vi "ZK Create MB.vi"() -> ()   [LabVIEW 2016, in "质控单元V1.lvlib"]
uses:
  <vilib>/Plasmionique/MB Master/MB_Master_Serial/MB_Master_Serial.lvclass
  D:/Program Files (x86)/National Instruments/LabVIEW 2016/vi.lib/Plasmionique/MB Master/MB_Master/MB_Master.lvclass
  <vilib>/Plasmionique/MB Master/MB_Master_TCP/MB_Master_TCP.lvclass
  <vilib>/Plasmionique/MB Master/MB_Master/MB_Master.lvclass
panel:
  out "auto connected":bool=TRUE
  out "error out":errorcluster
  out "Connected":bool
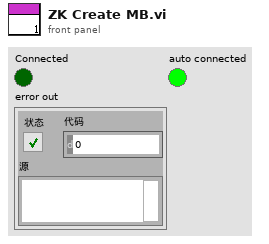
[diagram p1: front panel]
types:
  T1 = cluster{"baud rate (bps)":u32, "stop bits":u16, "parity":u16, "flow control":u16, "timeout":u32, "retries":i32}
  T2 = typedef "质控单元V1.lvlib/质控slave id.ctl" = enum16{"null", "氨氮", "总磷", "CODMn", "CODCr", "总氮"}
  T3 = cluster{"氨氮":bool, "总磷":bool, "总氮":bool, "CODMn":bool, "CODCr":bool, "氨氮总磷":bool, "总磷总氮":bool}
  T4 = typedef "质控单元V1.lvlib/质控仪器状态显示.ctl" = cluster{"运行模式":string, "运行状态":string, "液位状态":string, "告警状态":string, "加标体积":string}
  T5 = typedef "质控单元V1.lvlib/质控仪器状态.ctl" = cluster{"运行状态":T6, "加标体积":sgl, "NC":dbl, "液位状态":enum16{"无感应", "有感应"}, "告警状态":enum16{"无告警", "超时告警"}}
  T6 = typedef "质控单元V1.lvlib/质控运行状态.ctl" = enum16{"待机", "润洗", "进样", "加标", "排液", "搅拌", "超时告警"}
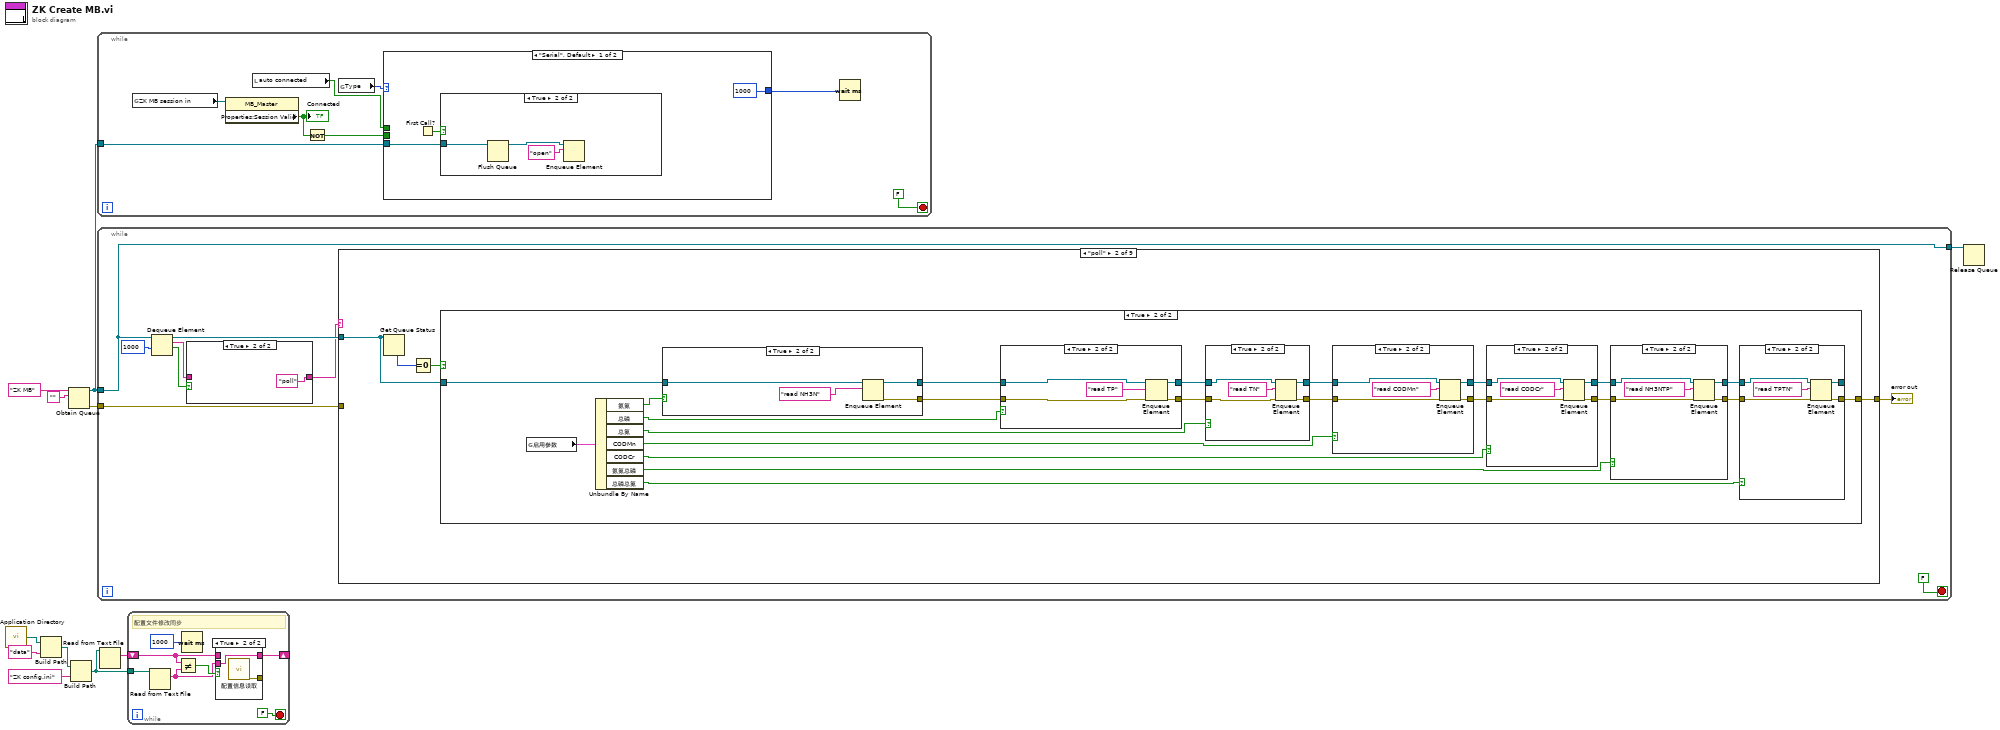
[diagram p0: block diagram]
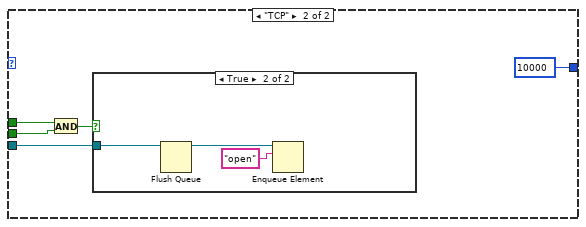
[diagram p4: hidden frame]
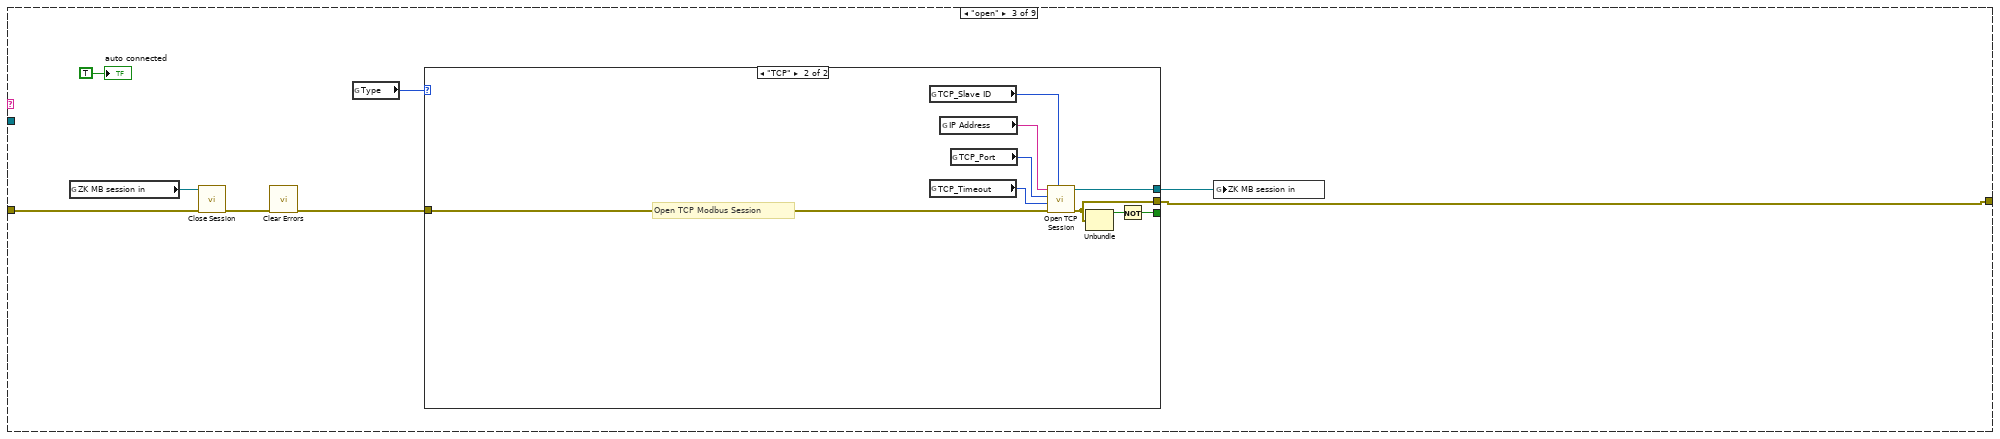
[diagram p16: hidden frame]
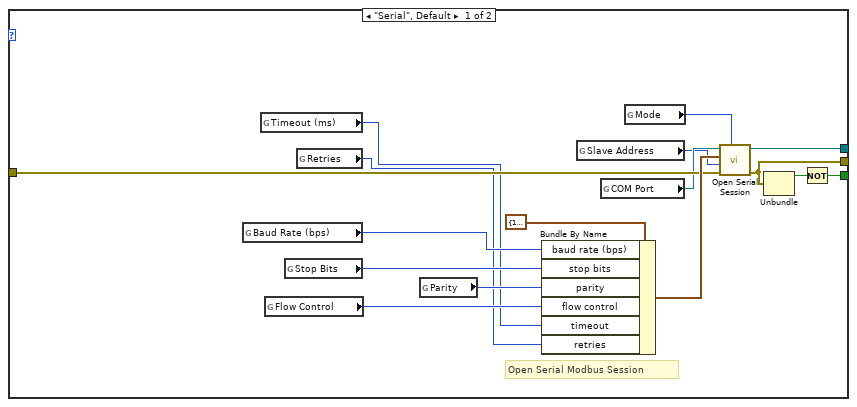
[diagram p17: hidden frame]
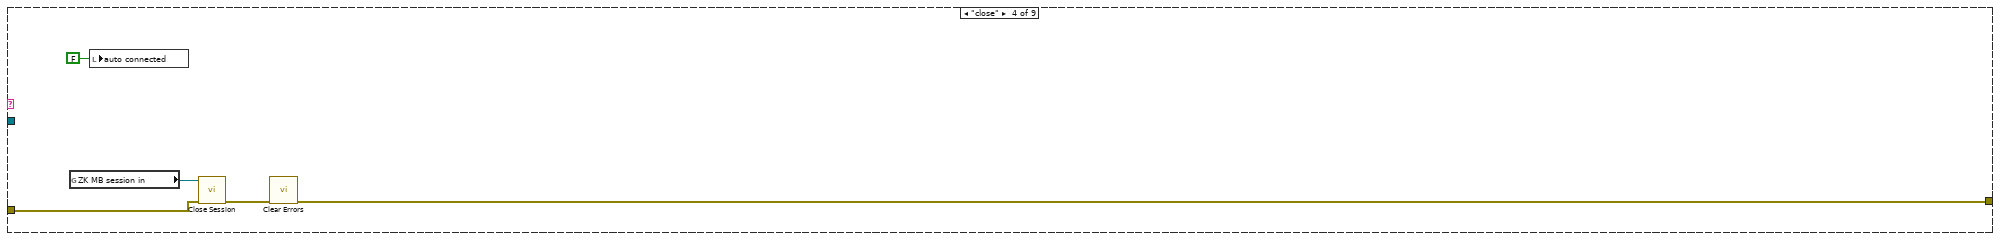
[diagram p18: hidden frame]
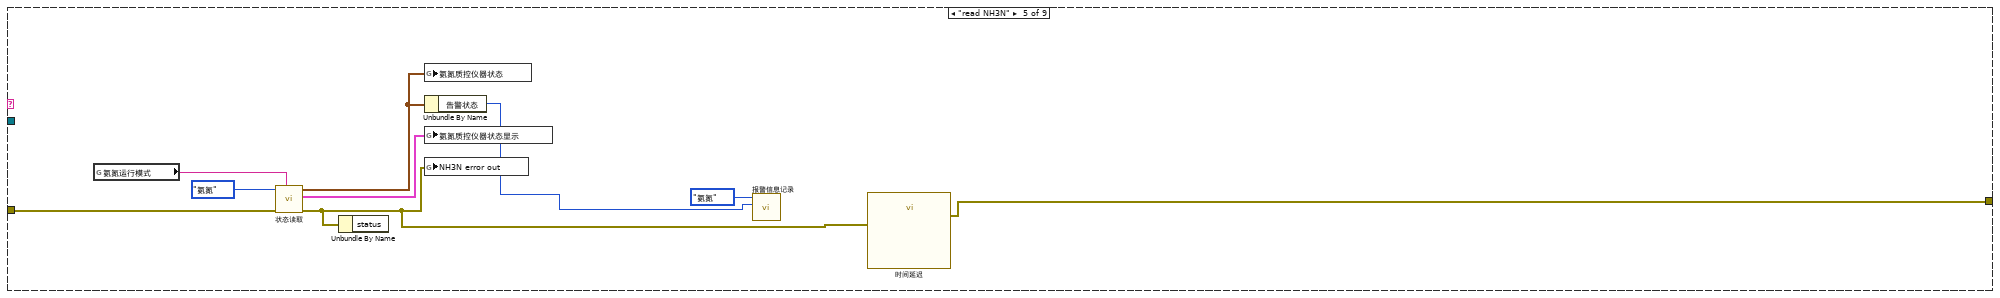
[diagram p19: hidden frame]
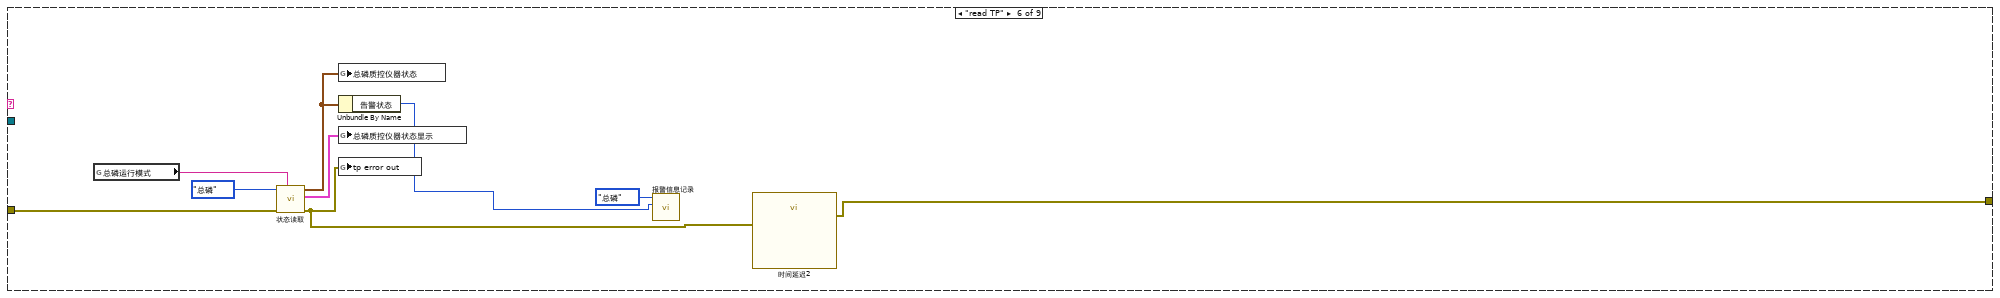
[diagram p20: hidden frame]
diagram:
  n1 = call <vilib>:"Application Directory.vi"() -> ("Application Directory"=w6:path)
  n2 = Build Path(base path=w6, name or relative path="data" ("名称或相对路径")) -> (appended path=w3:path)
  n3 = Obtain Queue(name (unnamed)="ZK MB" ("名称（未命名）"), element data type="") -> (queue out=w9:refnum<queue>, error out=w7:errorcluster)  [unwired: 3 in, 1 out]
  n4 = Build Path(base path=w3, name or relative path="ZK config.ini" ("名称或相对路径")) -> (appended path=w1:path)
  n5 = while {
    tunnel: w9 -> [w18]
    stop <- FALSE stop-if-true
    n6 = global read "ZK非断电保存全局变量.vi" "ZK MB session in"() -> (w15:refnum<class "MB_Master.lvclass">)
    n7 = property class="MB_Master"(reference=w15) -> ("Properties:Session Valid"=w14:bool)  [unwired: 1 in, 2 out]
    "Connected" <- w14
    n8 = local read "auto connected"() -> (w13:bool)
    n9 = Not(x=w14) -> (.not. x?=w12:bool)
    n10 = global read "ZK断电保存全局变量.vi" "Type"() -> (w19:enum16{"Serial", "TCP"})
    n11 = case shown="\"Serial\", Default" w19 {
      tunnel: w18 -> [w22 w30]
      tunnel: [u32 1000 ("等待时间（毫秒）") u32 10000 ("等待时间（毫秒）")] -> w16
      tunnel: w12 -> [_ w28]
      tunnel: w13 -> [_ w26]
      frame "Serial", Default {
        n12 = First Call?() -> (First Call?: T/F=w21:bool)
        n13 = case shown="True" w21 {
          tunnel: w22 -> [_ w25]
          frame False {
          }
          frame True {
            n14 = Flush Queue(queue=w25) -> (queue out=w23:refnum<queue>)  [unwired: 1 in, 2 out]
            n15 = Enqueue Element(queue=w23, element="open") -> ()  [unwired: 2 in, 3 out]
          }
        }
      }
      frame "TCP" {
        n16 = And(x=w26, y=w28) -> (x .and. y?=w27:bool)
        n17 = case shown="True" w27 {
          tunnel: w30 -> [_ w32]
          frame False {
          }
          frame True {
            n18 = Flush Queue(queue=w32) -> (queue out=w31:refnum<queue>)  [unwired: 1 in, 2 out]
            n19 = Enqueue Element(queue=w31, element="open") -> ()  [unwired: 2 in, 3 out]
          }
        }
      }
    }
    n20 = Wait (ms)(milliseconds to wait=w16) -> ()  [unwired: 1 out]
  }
  n21 = while {
    tunnel: w9 -> [w39]
    tunnel: [w39] -> w8
    tunnel: w7 -> [w34]
    stop <- FALSE stop-if-true
    n22 = Dequeue Element(queue=w39, timeout in ms (-1)=1000 ("超时毫秒(-1)")) -> (queue out=w40:refnum<queue>, element=w36:string, timed out?=w37:bool)  [unwired: 1 in, 1 out]
    n23 = case shown="True" w37 {
      tunnel: w36 -> [w43 _]
      tunnel: [w43 "poll"] -> w35
      frame False {
      }
      frame True {
      }
    }
    n24 = case shown="\"poll\"" w35 {
      tunnel: [w45 w49 w121 w154 w163 w173 w182 w190 w199] -> w41
      tunnel: w34 -> [w45 _ w120 w155 w165 w174 w183 w192 w201]
      tunnel: w40 -> [_ w48 _ _ _ _ _ _ _]
      frame Default {
      }
      frame "poll" {
        n25 = Get Queue Status(queue=w48) -> (# elements in queue=w47:i32)  [unwired: 2 in, 7 out]
        n26 = Equal To 0?(x=w47) -> (x = 0?=w46:bool)
        n27 = case shown="True" w46 {
          tunnel: [_ w55] -> w49
          tunnel: w48 -> [_ w50]
          frame False {
          }
          frame True {
            n28 = global read "ZK断电保存全局变量.vi" "启用参数"() -> (w63:T3)
            n29 = Unbundle By Name(w63) -> ("氨氮"=w62:bool, "总磷"=w61:bool, "总氮"=w60:bool, "CODMn"=w54:bool, "CODCr"=w53:bool, "氨氮总磷"=w52:bool, "总磷总氮"=w51:bool)
            n30 = case shown="True" w62 {
              tunnel: w50 -> [w114 w118]
              tunnel: [w114 w117] -> w71
              tunnel: [_ w116] -> w70
              frame False {
              }
              frame True {
                n31 = Enqueue Element(queue=w118, element="read NH3N") -> (queue out=w117:refnum<queue>, error out=w116:errorcluster)  [unwired: 2 in, 1 out]
              }
            }
            n32 = case shown="True" w61 {
              tunnel: w71 -> [w108 w113]
              tunnel: w70 -> [w107 w112]
              tunnel: [w108 w110] -> w69
              tunnel: [w107 w109] -> w66
              frame False {
              }
              frame True {
                n33 = Enqueue Element(queue=w113, element="read TP", error in (no error)=w112) -> (queue out=w110:refnum<queue>, error out=w109:errorcluster)  [unwired: 1 in, 1 out]
              }
            }
            n34 = case shown="True" w60 {
              tunnel: w69 -> [w101 w105]
              tunnel: [w101 w104] -> w59
              tunnel: w66 -> [w100 w103]
              tunnel: [w100 w102] -> w58
              frame False {
              }
              frame True {
                n35 = Enqueue Element(queue=w105, element="read TN", error in (no error)=w103) -> (queue out=w104:refnum<queue>, error out=w102:errorcluster)  [unwired: 1 in, 1 out]
              }
            }
            n36 = case shown="True" w54 {
              tunnel: w59 -> [w80 w84]
              tunnel: [w80 w83] -> w67
              tunnel: w58 -> [w79 w82]
              tunnel: [w79 w81] -> w64
              frame False {
              }
              frame True {
                n37 = Enqueue Element(queue=w84, element="read CODMn", error in (no error)=w82) -> (queue out=w83:refnum<queue>, error out=w81:errorcluster)  [unwired: 1 in, 1 out]
              }
            }
            n38 = case shown="True" w53 {
              tunnel: w67 -> [w73 w78]
              tunnel: w64 -> [w72 w77]
              tunnel: [w72 w75] -> w56
              tunnel: [w73 w74] -> w57
              frame False {
              }
              frame True {
                n39 = Enqueue Element(queue=w78, element="read CODCr", error in (no error)=w77) -> (queue out=w74:refnum<queue>, error out=w75:errorcluster)  [unwired: 1 in, 1 out]
              }
            }
            n40 = case shown="True" w52 {
              tunnel: w57 -> [w94 w98]
              tunnel: [w94 w97] -> w68
              tunnel: w56 -> [w93 w96]
              tunnel: [w93 w95] -> w65
              frame False {
              }
              frame True {
                n41 = Enqueue Element(queue=w98, element="read NH3NTP", error in (no error)=w96) -> (queue out=w97:refnum<queue>, error out=w95:errorcluster)  [unwired: 1 in, 1 out]
              }
            }
            n42 = case shown="True" w51 {
              tunnel: w68 -> [w87 w91]
              tunnel: [w87 w90] -> _
              tunnel: w65 -> [w86 w89]
              tunnel: [w86 w88] -> w55
              frame False {
              }
              frame True {
                n43 = Enqueue Element(queue=w91, element="read TPTN", error in (no error)=w89) -> (queue out=w90:refnum<queue>, error out=w88:errorcluster)  [unwired: 1 in, 1 out]
              }
            }
          }
        }
      }
      frame "open" {
        n44 = global read "ZK非断电保存全局变量.vi" "ZK MB session in"() -> (w123:refnum<class "MB_Master.lvclass">)
        n45 = call-dynamic "Close Session.vi"("error in (no error)"=w120, "MB session in"=w123) -> ("error out"=w125:errorcluster)  [unwired: 9 in]
        n46 = call <vilib>:"Clear Errors.vi"("error in (no error)"=w125) -> ("error out"=w126:errorcluster)  [unwired: 5 in, 1 out]
        n47 = global read "ZK断电保存全局变量.vi" "Type"() -> (w124:enum16{"Serial", "TCP"})
        n48 = case shown="\"TCP\"" w124 {
          tunnel: [w140 w147] -> w122
          tunnel: [w139 w148] -> w121
          tunnel: [w137 w149] -> _
          tunnel: w126 -> [w136 w151]
          frame "Serial", Default {
            # "Open Serial Modbus Session"
            n49 = global read "ZK断电保存全局变量.vi" "Baud Rate (bps)"() -> (w132:u32)
            n50 = global read "ZK断电保存全局变量.vi" "Timeout (ms)"() -> (w128:u32)
            n51 = global read "ZK断电保存全局变量.vi" "Flow Control"() -> (w129:u16)
            n52 = global read "ZK断电保存全局变量.vi" "Stop Bits"() -> (w131:u16)
            n53 = global read "ZK断电保存全局变量.vi" "Retries"() -> (w127:i32)
            n54 = global read "ZK断电保存全局变量.vi" "Parity"() -> (w130:u16)
            n55 = Bundle By Name(cluster=T1 {"baud rate (bps)"=19200, "stop bits"=10, "parity"=0, "flow control"=0, "timeout"=1000, "retries"=1} ("Serial Config"), "baud rate (bps)"=w132, "stop bits"=w131, "parity"=w130, "flow control"=w129, "timeout"=w128, "retries"=w127) -> (w141:T1)
            n56 = global read "ZK断电保存全局变量.vi" "Slave Address"() -> (w133:u8)
            n57 = global read "ZK断电保存全局变量.vi" "COM Port"() -> (w134:refnum<visa-resource-name>)
            n58 = global read "ZK断电保存全局变量.vi" "Mode"() -> (w135:enum16{"RTU", "ASCII"})
            n59 = call <vilib>:"Open Serial Session.vi"("Mode (RTU)"=w135, "Error in"=w136, "Slave ID"=w133, "Serial Config"=w141, "VISA Resource"=w134) -> ("Error out"=w139:errorcluster, "MB_Serial session"=w140:refnum<class "MB_Master_Serial.lvclass">)  [unwired: 5 in]
            n60 = Unbundle(w139) -> ("status"=w138:bool)  [unwired: 2 out]
            n61 = Not(x=w138) -> (.not. x?=w137:bool)
          }
          frame "TCP" {
            # "Open TCP Modbus Session"
            n62 = global read "ZK断电保存全局变量.vi" "TCP_Slave ID"() -> (w146:u8)
            n63 = global read "ZK断电保存全局变量.vi" "TCP_Timeout"() -> (w143:i32)
            n64 = global read "ZK断电保存全局变量.vi" "IP Address"() -> (w145:string)
            n65 = global read "ZK断电保存全局变量.vi" "TCP_Port"() -> (w144:u16)
            n66 = call <vilib>:"Open TCP Session.vi"("Slave ID (255)"=w146, "error in (no error)"=w151, "Timeout (10000)"=w143, "Port (502)"=w144, "IP Address"=w145) -> ("error out"=w148:errorcluster, "MB_TCP session"=w147:refnum<class "MB_Master_TCP.lvclass">)  [unwired: 5 in]
            n67 = Unbundle(w148) -> ("status"=w150:bool)  [unwired: 2 out]
            n68 = Not(x=w150) -> (.not. x?=w149:bool)
          }
        }
        n69 = global write "ZK非断电保存全局变量.vi" "ZK MB session in"(w122) -> ()
        "auto connected" <- TRUE
      }
      frame "close" {
        n70 = global read "ZK非断电保存全局变量.vi" "ZK MB session in"() -> (w153:refnum<class "MB_Master.lvclass">)
        n71 = local write "auto connected"(FALSE ("auto connected")) -> ()
        n72 = call-dynamic "Close Session.vi"("error in (no error)"=w155, "MB session in"=w153) -> ("error out"=w156:errorcluster)  [unwired: 9 in]
        n73 = call <vilib>:"Clear Errors.vi"("error in (no error)"=w156) -> ("error out"=w154:errorcluster)  [unwired: 5 in, 1 out]
      }
      frame "read NH3N" {
        n74 = global read "ZK非断电保存全局变量.vi" "氨氮运行模式"() -> (w160:string)
        n75 = call "状态读取.vi"("运行模式"=w160, "error in (no error)"=w165, "Slave ID"=质控slave_id."氨氮") -> ("error out"=w158:errorcluster, "质控仪器状态显示"=w162:T4, "质控仪器状态"=w161:T5)  [unwired: 6 in]
        n76 = Unbundle By Name(w158) -> ()  [unwired: 1 out]
        n77 = global write "ZK非断电保存全局变量.vi" "氨氮质控仪器状态"(w161) -> ()
        n78 = Unbundle By Name(w161) -> ("告警状态"=w157:enum16{"无告警", "超时告警"})
        n79 = global write "ZK非断电保存全局变量.vi" "氨氮质控仪器状态显示"(w162) -> ()
        n80 = global write "ZK非断电保存全局变量.vi" "NH3N error out"(w158) -> ()
        n81 = call "报警信息记录.vi"("CODE"=w157, "Slave ID"=质控slave_id."氨氮") -> ()  [unwired: 9 in, 1 out]
        n82 = call "时间延迟"("error in (no error)"=w158) -> ("error out"=w163:errorcluster)  [unwired: 10 in]
      }
      frame "read TP" {
        n83 = global read "ZK非断电保存全局变量.vi" "总磷运行模式"() -> (w170:string)
        n84 = call "状态读取.vi"("运行模式"=w170, "error in (no error)"=w174, "Slave ID"=质控slave_id."总磷") -> ("error out"=w167:errorcluster, "质控仪器状态显示"=w172:T4, "质控仪器状态"=w171:T5)  [unwired: 6 in]
        n85 = global write "ZK非断电保存全局变量.vi" "总磷质控仪器状态"(w171) -> ()
        n86 = Unbundle By Name(w171) -> ("告警状态"=w166:enum16{"无告警", "超时告警"})
        n87 = global write "ZK非断电保存全局变量.vi" "总磷质控仪器状态显示"(w172) -> ()
        n88 = global write "ZK非断电保存全局变量.vi" "tp error out"(w167) -> ()
        n89 = call "报警信息记录.vi"("CODE"=w166, "Slave ID"=质控slave_id."总磷") -> ()  [unwired: 9 in, 1 out]
        n90 = call "时间延迟2"("error in (no error)"=w167) -> ("error out"=w173:errorcluster)  [unwired: 10 in]
      }
      frame "read TN" {
        n91 = global read "ZK非断电保存全局变量.vi" "总氮运行模式"() -> (w179:string)
        n92 = call "状态读取.vi"("运行模式"=w179, "error in (no error)"=w183, "Slave ID"=质控slave_id."总氮") -> ("error out"=w176:errorcluster, "质控仪器状态显示"=w181:T4, "质控仪器状态"=w180:T5)  [unwired: 6 in]
        n93 = global write "ZK非断电保存全局变量.vi" "总氮质控仪器状态"(w180) -> ()
        n94 = Unbundle By Name(w180) -> ("告警状态"=w175:enum16{"无告警", "超时告警"})
        n95 = global write "ZK非断电保存全局变量.vi" "总氮质控仪器状态显示"(w181) -> ()
        n96 = global write "ZK非断电保存全局变量.vi" "tn error out"(w176) -> ()
        n97 = call "报警信息记录.vi"("CODE"=w175, "Slave ID"=质控slave_id."总氮") -> ()  [unwired: 9 in, 1 out]
        n98 = call "时间延迟3"("error in (no error)"=w176) -> ("error out"=w182:errorcluster)  [unwired: 10 in]
      }
      frame "read CODMn" {
        n99 = global read "ZK非断电保存全局变量.vi" "CODMn运行模式"() -> (w187:string)
        n100 = call "状态读取.vi"("运行模式"=w187, "error in (no error)"=w192, "Slave ID"=质控slave_id."CODMn") -> ("error out"=w185:errorcluster, "质控仪器状态显示"=w189:T4, "质控仪器状态"=w188:T5)  [unwired: 6 in]
        n101 = Unbundle By Name(w188) -> ("告警状态"=w184:enum16{"无告警", "超时告警"})
        n102 = global write "ZK非断电保存全局变量.vi" "CODMn质控仪器状态"(w188) -> ()
        n103 = global write "ZK非断电保存全局变量.vi" "CODMn质控仪器状态显示"(w189) -> ()
        n104 = global write "ZK非断电保存全局变量.vi" "CODMn error out"(w185) -> ()
        n105 = call "报警信息记录.vi"("CODE"=w184, "Slave ID"=质控slave_id."CODMn") -> ()  [unwired: 9 in, 1 out]
        n106 = call "时间延迟4"("error in (no error)"=w185) -> ("error out"=w190:errorcluster)  [unwired: 10 in]
      }
      frame "read CODCr" {
        n107 = global read "ZK非断电保存全局变量.vi" "CODCr运行模式"() -> (w196:string)
        n108 = call "状态读取.vi"("运行模式"=w196, "error in (no error)"=w201, "Slave ID"=质控slave_id."CODCr") -> ("error out"=w194:errorcluster, "质控仪器状态显示"=w198:T4, "质控仪器状态"=w197:T5)  [unwired: 6 in]
        n109 = Unbundle By Name(w194) -> ()  [unwired: 1 out]
        n110 = Unbundle By Name(w197) -> ("告警状态"=w193:enum16{"无告警", "超时告警"})
        n111 = global write "ZK非断电保存全局变量.vi" "CODCr质控仪器状态"(w197) -> ()
        n112 = global write "ZK非断电保存全局变量.vi" "CODcr质控仪器状态显示"(w198) -> ()
        n113 = global write "ZK非断电保存全局变量.vi" "CODCr error out"(w194) -> ()
        n114 = call "报警信息记录.vi"("CODE"=w193, "Slave ID"=质控slave_id."CODCr") -> ()  [unwired: 9 in, 1 out]
        n115 = call "时间延迟5"("error in (no error)"=w194) -> ("error out"=w199:errorcluster)  [unwired: 10 in]
      }
    }
    "error out" <- w41
  }
  n116 = Read from Text File(file (use dialog)=w1) -> (text=w2:string)  [unwired: 3 in, 3 out]
  n117 = while {
    shift-right: [w206] -> _
    shift-left: w2 -> [w204]
    tunnel: w1 -> [w208]
    stop <- FALSE stop-if-true
    # "配置文件修改同步"
    n118 = Read from Text File(file (use dialog)=w208) -> (text=w205:string)  [unwired: 3 in, 3 out]
    n119 = Not Equal?(x=w204, y=w205) -> (x != y?=w207:bool)
    n120 = Wait (ms)(milliseconds to wait=u32 1000 ("等待时间（毫秒）")) -> ()  [unwired: 1 out]
    n121 = case shown="True" w207 {
      tunnel: [w209 w211] -> w206
      tunnel: w205 -> [_ w211]
      tunnel: w204 -> [w209 _]
      tunnel: [_ w210] -> _
      frame False {
      }
      frame True {
        n122 = call "配置信息读取.vi"() -> ("error out"=w210:errorcluster)  [unwired: 11 in]
      }
    }
  }
  n123 = Release Queue(queue=w8) -> ()  [unwired: 2 in, 3 out]
